vi "Sort Items.vi"(1 "Component Type":T1, 2 "Unsorted Componet In":T2[](array[typedef])) -> (0 "Sorted Component Array Out":T2[](array[typedef]))   [LabVIEW 2013]
uses:
  Controls/Display Component Line.ctl
  Controls/Components.ctl
  Controls/Component Sub Type.ctl
  Controls/Add Button.ctl
  Controls/Subtract Button.ctl
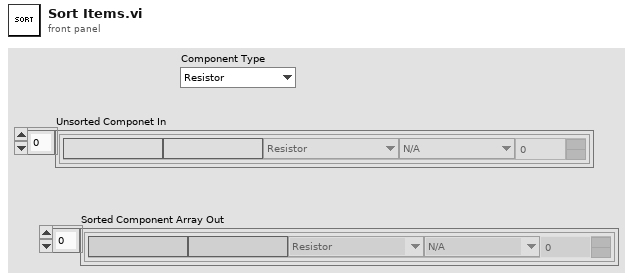
[diagram p1: front panel]
types:
  T1 = typedef "Components.ctl" = enum16{"Resistor", "Capacitor", "Diode", "Voltage Regulator", "Transistors", "ICs", "Misc"}
  T2 = typedef "Display Component Line.ctl" = cluster{"Part Number":string, "Code (Value)":string, "Component Type":T1, "Component Subtype":T3, "Quantity":u32, "Add":T4, "Subtract":T5}
  T3 = typedef "Component Sub Type.ctl" = enum16{"N/A", "Carbon", "Variable - Trimmer", "Variable - Pot", "Ceramic", "Electrolitic", "Zenner", "TO-92", "TO-220", "NPN", "PNP", "CMOS", "Processor"}
  T4 = typedef "Add Button.ctl" = bool
  T5 = typedef "Subtract Button.ctl" = bool
  T6 = cluster{"Numeric":dbl, "Part Number":string, "Component Type":T1, "Component Subtype":T3, "Quantity":u32, "Code (Value)":string}[]
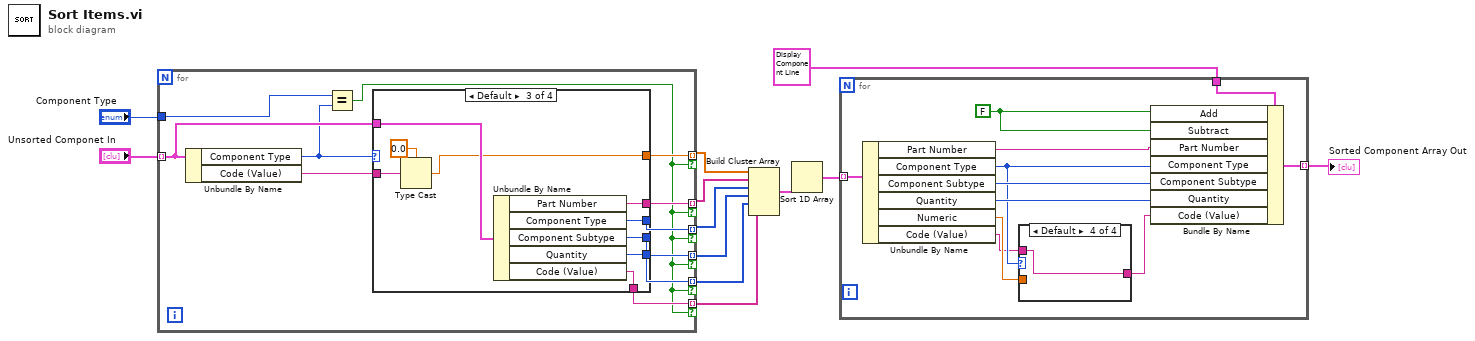
[diagram p0: block diagram]
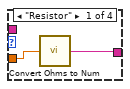
[diagram p2: hidden frame]
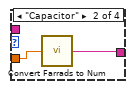
[diagram p3: hidden frame]
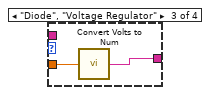
[diagram p4: hidden frame]
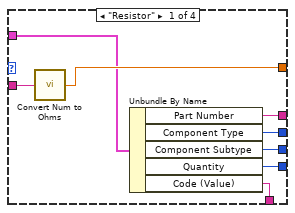
[diagram p5: hidden frame]
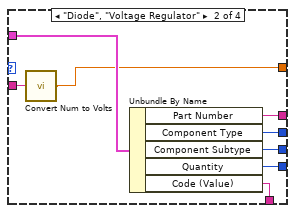
[diagram p6: hidden frame]
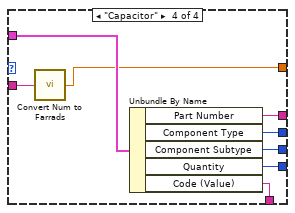
[diagram p7: hidden frame]
diagram:
  n1 = for {
    tunnel: "Unsorted Componet In" -> [w22] mode=indexing
    tunnel: [w21] -> w4 mode=indexing if=w13
    tunnel: [w20] -> w5 mode=indexing if=w13
    tunnel: [w19] -> w8 mode=indexing if=w13
    tunnel: [w18] -> w9 mode=indexing if=w13
    tunnel: [w17] -> w10 mode=indexing if=w13
    tunnel: "Component Type" -> [w15]
    tunnel: [w14] -> w1 mode=indexing if=w13
    n2 = Unbundle By Name(w22) -> ("Component Type"=w16:T1, "Code (Value)"=w23:string)
    n3 = Equal?(x=w15, y=w16) -> (x = y?=w13:bool)
    n4 = case shown="Default" w16 {
      tunnel: w23 -> [w31 w34 w42 w51]
      tunnel: w22 -> [w29 w39 w48 w56]
      tunnel: [w30 w33 w40 w50] -> w21
      tunnel: [w28 w38 w47 w55] -> w20
      tunnel: [w27 w37 w46 w54] -> w19
      tunnel: [w26 w36 w45 w53] -> w18
      tunnel: [w25 w35 w44 w52] -> w17
      tunnel: [w24 w32 w43 w49] -> w14
      frame "Resistor" {
        n5 = call "Convert Num to Ohms.vi"("String"=w31) -> ("Numeric"=w30:dbl)
        n6 = Unbundle By Name(w29) -> ("Part Number"=w28:string, "Component Type"=w27:T1, "Component Subtype"=w26:T3, "Quantity"=w25:u32, "Code (Value)"=w24:string)
      }
      frame "Diode", "Voltage Regulator" {
        n7 = call "Convert Num to Volts.vi"("String"=w34) -> ("Numeric"=w33:dbl)
        n8 = Unbundle By Name(w39) -> ("Part Number"=w38:string, "Component Type"=w37:T1, "Component Subtype"=w36:T3, "Quantity"=w35:u32, "Code (Value)"=w32:string)
      }
      frame Default {
        n9 = Type Cast(type=0.0 ("Numeric"), x=w42) -> (*(type *) &x=w40:dbl)
        n10 = Unbundle By Name(w48) -> ("Part Number"=w47:string, "Component Type"=w46:T1, "Component Subtype"=w45:T3, "Quantity"=w44:u32, "Code (Value)"=w43:string)
      }
      frame "Capacitor" {
        n11 = call "Convert Num to Farrads.vi"("String"=w51) -> ("Numeric"=w50:dbl)
        n12 = Unbundle By Name(w56) -> ("Part Number"=w55:string, "Component Type"=w54:T1, "Component Subtype"=w53:T3, "Quantity"=w52:u32, "Code (Value)"=w49:string)
      }
    }
  }
  n13 = Build Cluster Array(w4, w5, w8, w9, w10, w1) -> (w6:T6)
  n14 = Sort 1D Array(array=w6) -> (sorted array=w7:T6)
  n15 = for {
    tunnel: w7 -> [w67] mode=indexing
    tunnel: T2 {"Part Number"="", "Code (Value)"="", "Component Type"=enum."Voltage Regulator", "Component Subtype"=enum."N/A", "Quantity"=0, "Add"=FALSE, "Subtract"=FALSE} ("Display Components Line") -> [w66]
    tunnel: [w61] -> w12 mode=indexing
    w62 = FALSE
    n16 = Unbundle By Name(w67) -> ("Part Number"=w65:string, "Component Type"=w60:T1, "Component Subtype"=w64:T3, "Quantity"=w63:u32, "Numeric"=w59:dbl, "Code (Value)"=w57:string)
    n17 = case shown="Default" w60 {
      tunnel: w59 -> [w69 w71 w73 _]
      tunnel: [w68 w70 w72 w74] -> w58
      tunnel: w57 -> [_ _ _ w74]
      frame "Resistor" {
        n18 = call "Convert Ohms to Num.vi"("Numeric"=w69) -> ("String"=w68:string)
      }
      frame "Capacitor" {
        n19 = call "Convert Farrads to Num.vi"("Numeric"=w71) -> ("String"=w70:string)
      }
      frame "Diode", "Voltage Regulator" {
        n20 = call "Convert Volts to Num.vi"("Numeric"=w73) -> ("String"=w72:string)
      }
      frame Default {
      }
    }
    n21 = Bundle By Name(cluster=w66, "Add"=w62, "Subtract"=w62, "Part Number"=w65, "Component Type"=w60, "Component Subtype"=w64, "Quantity"=w63, "Code (Value)"=w58) -> (w61:T2)
  }
  "Sorted Component Array Out" <- w12
